vi "main.vi"() -> ()   [LabVIEW 2018]
uses:
  <vilib>/addons/database/Connection.llb/DB Tools Open Connec (Path).vi
  <vilib>/addons/database/NI_Database_API.lvlib
panel:
  out "负责人信息":T1
  out "疫苗信息":T2 {"生产日期" format="%<%Y/%m/%d>T"}
  in  "CYJ":bool
  in  "比例尺":i16(slide) scale=6.0..18.0
  in  "地图":refnum<k7>(container) caption="网页浏览器"
  out "掉线":bool
  out "经度":string
  out "纬度":string
  out "数据":bool
  in  "stop":bool caption="停止"
  out "时间":timestamp format="%<%x %H:%M:%S>T"
  out "温度":dbl format="%#.1g"
  out "id":i16
  out "定位":bool
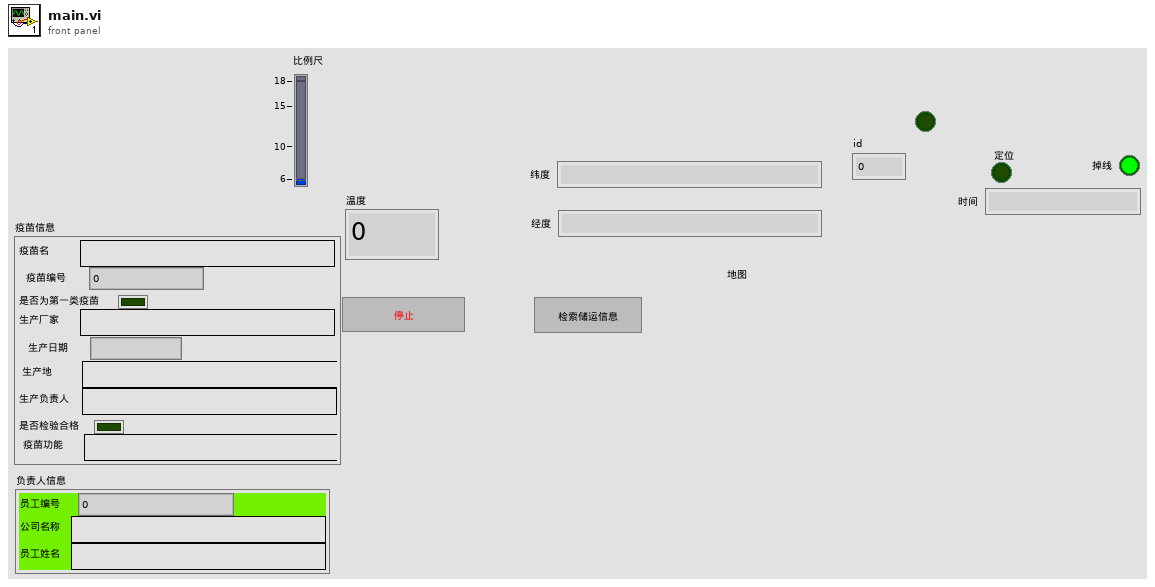
[diagram p1: front panel]
types:
  T1 = typedef "人员信息.ctl" = cluster{"员工编号":i32, "公司名称":string, "员工姓名":string}
  T2 = typedef "疫苗信息.ctl" = cluster{"疫苗名":string, "疫苗编号":i32, "是否为第一类疫苗":bool, "生产厂家":string, "生产日期":timestamp, "生产地":string, "生产负责人":string, "是否检验合格":bool, "疫苗功能":string}
  T3 = typedef "NI_Database_API.lvlib/Conn ObjectReference.ctl" = refnum<k1>
  T4 = typedef "储运信息.ctl" = cluster{"纬度":sgl, "经度":sgl, "温度":sgl, "负责人":i32, "区域":string, "记录时间":timestamp}
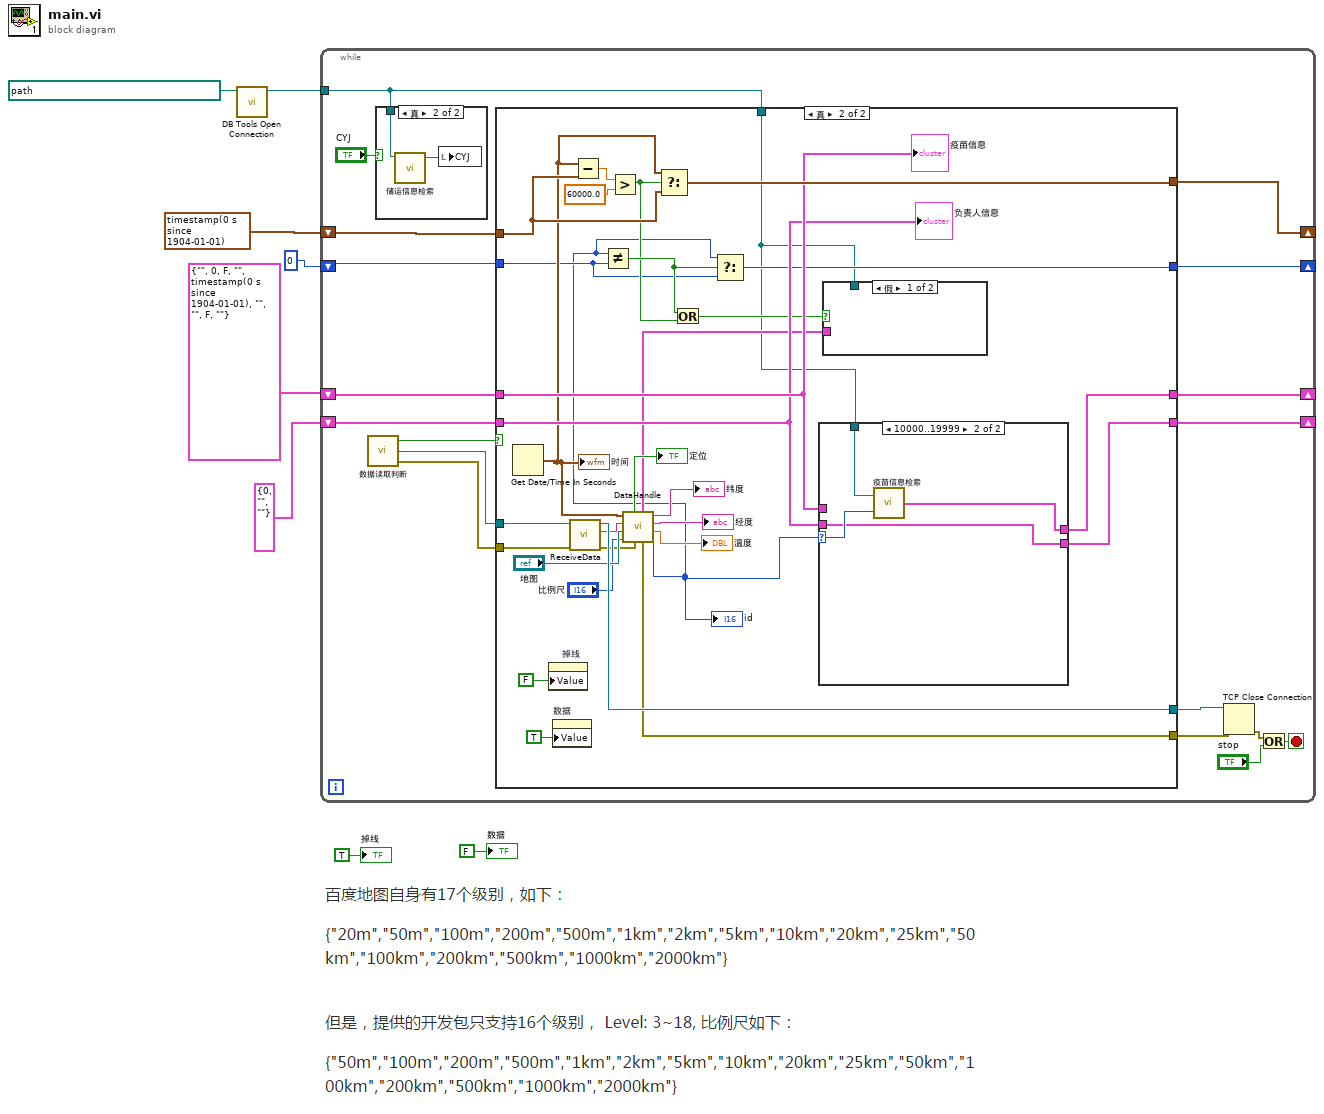
[diagram p0: block diagram]
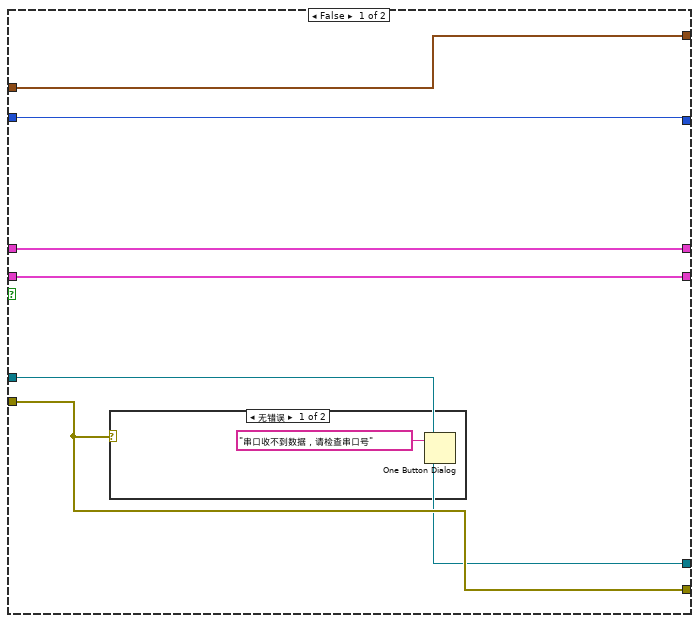
[diagram p3: hidden frame]
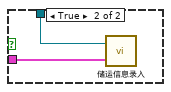
[diagram p5: hidden frame]
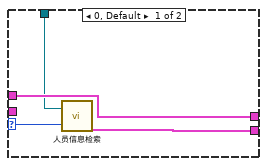
[diagram p6: hidden frame]
diagram:
  n1 = call-poly <vilib>:"DB Tools Open Connection.vi"("connection information"=path "D:/2019毕业设计/Code/GPData.udl" ("路径")) -> ("connection reference"=w6:T3)  [unwired: 7 in, 1 out]
  n2 = while {
    tunnel: w6 -> [w12]
    shift-right: [w11] -> _
    shift-left: T2 {"疫苗名"="", "疫苗编号"=0, "是否为第一类疫苗"=FALSE, "生产厂家"="", "生产日期"=timestamp(0 s since 1904-01-01), "生产地"="", "生产负责人"="", "是否检验合格"=FALSE, "疫苗功能"=""} ("簇") -> [w17]
    shift-right: [w15] -> _
    shift-left: T1 {"员工编号"=0, "公司名称"="", "员工姓名"=""} ("负责人数据") -> [w16]
    shift-right: [w13] -> _
    shift-left: timestamp(0 s since 1904-01-01) ("时间标识") -> [w14]
    shift-right: [w9] -> _
    shift-left: 0 -> [w10]
    stop <- w26 stop-if-true
    n3 = call "数据读取判断.vi"() -> ("error out"=w22:errorcluster, "connection ID"=w23:refnum<k5>, "判断错误"=w24:bool)
    n4 = case shown="真" "CYJ" {
      tunnel: w12 -> [_ w28]
      frame False {
      }
      frame True {
        n5 = call "储运信息检索.vi"("connection reference"=w28) -> ("布尔"=w27:bool)  [unwired: 3 in, 2 out]
        n6 = local write "CYJ"(w27) -> ()
      }
    }
    n7 = case shown="真" w24 {
      tunnel: w22 -> [w34 w65]
      tunnel: [w33 w64] -> w19
      tunnel: [w34 w43] -> w21
      tunnel: w23 -> [w33 w63]
      tunnel: w12 -> [_ w36]
      tunnel: [w32 w61] -> w11
      tunnel: w17 -> [w32 w55]
      tunnel: w16 -> [w31 w54]
      tunnel: [w31 w60] -> w15
      tunnel: w14 -> [w30 w57]
      tunnel: [w30 w56] -> w13
      tunnel: w10 -> [w29 w38]
      tunnel: [w29 w53] -> w9
      frame False {
        n8 = case shown="无错误" w34 {
          frame No Error {
            n9 = One Button Dialog(message="串口收不到数据，请检查串口号" ("消息")) -> ()  [unwired: 1 in, 1 out]
          }
          frame Error {
          }
        }
      }
      frame True {
        n10 = Get Date/Time In Seconds() -> (seconds since 1Jan1904=w48:timestamp)
        "时间" <- w48
        n11 = property on="掉线" class="Bool (严格)"("Value"=FALSE ("掉线")) -> ()  [unwired: 2 in, 2 out]
        n12 = property on="数据" class="Bool (严格)"("Value"=TRUE ("状态")) -> ()  [unwired: 2 in, 2 out]
        n13 = call "ReceiveData.vi"("错误输入（无错误）"=w65, "连接ID"=w63) -> ("错误输出"=w44:errorcluster, "dataOut"=w47:string, "连接ID输出"=w64:refnum<k5>)  [unwired: 5 in, 2 out]
        n14 = Subtract(x=w48, y=w57) -> (x-y=w59:dbl)
        n15 = Greater?(x=w59, y=60000.0) -> (0:w51:bool)
        n16 = call "DataHandle.vi"("error IO"=w44, "滑动杆"="比例尺", "地图"="地图", "data"=w47, "时间"=w48) -> ("uid"=w37:i16, "温度"=→"温度":sgl, "经度显示"=→"经度":string, "纬度显示"=→"纬度":string, "错误输出"=w43:errorcluster, "储运信息簇"=w39:T4, "定位"=→"定位":bool)
        "id" <- w37
        n17 = Not Equal?(x=w37, y=w38) -> (x != y?=w52:bool)
        n18 = Select(t=w48, s=w51, f=w57) -> (s? t:f=w56:timestamp)
        n19 = Or(x=w52, y=w51) -> (x .or. y?=w50:bool)
        n20 = Select(t=w37, s=w52, f=w38) -> (s? t:f=w53:i32)
        n21 = case shown="10000..19999" w37 {
          selector: w37 -> [w72 w76]
          tunnel: [w71 w75] -> w61
          tunnel: w55 -> [w71 _]
          tunnel: w54 -> [_ w74]
          tunnel: [w70 w74] -> w60
          tunnel: w36 -> [w69 w73]
          frame 0, Default {
            n22 = call "人员信息检索.vi"("工作人员编号"=w72, "connection reference"=w69) -> ("负责人数据"=w70:T1)
          }
          frame 10000..19999 {
            n23 = call "疫苗信息检索.vi"("疫苗编号"=w76, "connection reference"=w73) -> ("疫苗数据"=w75:T2)
          }
        }
        n24 = case shown="假" w50 {
          tunnel: w36 -> [_ w68]
          tunnel: w39 -> [_ w67]
          frame False {
          }
          frame True {
            n25 = call "储运信息录入.vi"("簇"=w67, "connection reference"=w68) -> ()  [unwired: 1 out]
          }
        }
        "疫苗信息" <- w55
        "负责人信息" <- w54
      }
    }
    n26 = TCP Close Connection(connection ID=w19, error in (no error)=w21) -> (error out=w25:errorcluster)  [unwired: 1 in, 1 out]
    n27 = Or(x=w25, y="stop") -> (x .or. y?=w26:bool)
  }
  "掉线" <- TRUE ("掉线")
  "数据" <- FALSE ("串口")
